vi "Enum To String Method.vi"() -> ()   [LabVIEW 2020]
uses:
  <userlib>/_NEVSTOP/Communicable State Machine(CSM)/_Support/Typedef/_CSM_GlobalLog_MSG_TYPE.ctl
  <userlib>/_NEVSTOP/Communicable State Machine(CSM)/Communicable State Machine.lvlib
panel:
  out "inside 3":i32=999
  out "inside 2":i32=999
  out "inside":i32=999
  out "outside":i32=199
  out "unit (ms)":dbl[][](graph)=[[0.0, 0.0, 0.0, 0.0, 0.0, 0.0, 0.0, 0.0, 0.0, 0.0, 0.0, 0.0, 0.0, 0.0, 0.0, 0.0, 0.0, 0.0, 0.0, 0.0, 0.0, 0.0, 0.0, 0.0, 0.0, 0.0, 0.0, 0.0, 0.0, 0.0, 0.0, 0.0, 0.0, 0.0, 0.0, 0.0, 0.0, 0.0, 0.0, 0.001, 0.0, 0.001, 0.0, 0.0, 0.0, 0.0, 0.0, 0.001, 0.0, 0.0, 0.0, 0.0, 0.0, 0.0, 0.0, 0.0, 0.0, 0.0, 0.0, 0.0, 0.0, 0.0, 0.0, 0.0, 0.0, 0.0, 0.0, 0.0, 0.0, 0.001, 0.0, 0.0, 0.0, 0.0, 0.0, 0.0, 0.0, 0.0, 0.0, 0.0, 0.0, 0.0, 0.0, 0.0, 0.0, 0.0, 0.0, 0.0, 0.0, 0.0, 0.0, 0.0, 0.0, 0.0, 0.001, 0.0, 0.0, 0.0, 0.0, 0.0, 0.0, 0.0, 0.0, 0.0, 0.0, 0.0, 0.0, 0.0, 0.0, 0.0, 0.0, 0.0, 0.0, 0.0, 0.0, 0.0, 0.0, 0.001, 0.0, 0.0, 0.0, 0.0, 0.0, 0.0, 0.001, 0.0, 0.0, 0.0, 0.0, 0.0, 0.0, 0.0, 0.0, 0.0, 0.0, 0.0, 0.0, 0.0, 0.0, 0.0, 0.0, 0.001, 0.0, 0.0, 0.0, 0.0, 0.0, 0.0, 0.0, 0.0, 0.0, 0.0, 0.0, 0.0, 0.0, 0.0, 0.0, 0.0, 0.0, 0.0, 0.0, 0.0, 0.0, 0.0, 0.0, 0.001, 0.001, 0.001, 0.0, 0.0, 0.0, 0.0, 0.0, 0.0, 0.0, 0.001, 0.0, 0.0, 0.0, 0.0, 0.0, 0.0, 0.0, 0.0, 0.0, 0.0, 0.0, 0.0, 0.0, 0.0, 0.0, 0.0, 0.0, 0.0, 0.0, 0.0, 0.0, 0.0, 0.0, 0.0], [0.024, 0.012, 0.007, 0.009, 0.017, 0.007, 0.007, 0.008, 0.007, 0.017, 0.007, 0.009, 0.007, 0.025, 0.021, 0.021, 0.043, 0.037, 0.019, 0.008, 0.006, 0.007, 0.009, 0.007, 0.009, 0.008, 0.007, 0.008, 0.007, 0.008, 0.007, 0.018, 0.01, 0.008, 0.01, 0.008, 0.008, 0.009, 0.009, 0.007, 0.019, 0.007, 0.011, 0.008, 0.01, 0.009, 0.02, 0.009, 0.008, 0.01, 0.007, 0.013, 0.007, 0.007, 0.007, 0.008, 0.007, 0.02, 0.01, 0.007, 0.008, 0.009, 0.012, 0.007, 0.006, 0.009, 0.01, 0.013, 0.012, 0.013, 0.019, 0.01, 0.017, 0.014, 0.016, 0.039, 0.017, 0.018, 0.01, 0.017, 0.014, 0.028, 0.024, 0.031, 0.022, 0.018, 0.007, 0.022, 0.015, 0.016, 0.015, 0.014, 0.009, 0.013, 0.007, 0.014, 0.013, 0.007, 0.009, 0.009, 0.018, 0.008, 0.008, 0.008, 0.008, 0.009, 0.007, 0.009, 0.011, 0.021, 0.007, 0.012, 0.007, 0.009, 0.008, 0.009, 0.017, 0.009, 0.007, 0.008, 0.008, 0.008, 0.014, 0.008, 0.007, 0.009, 0.008, 0.021, 0.009, 0.018, 0.009, 0.011, 0.008, 0.009, 0.009, 0.008, 0.006, 0.011, 0.021, 0.015, 0.008, 0.017, 0.009, 0.008, 0.015, 0.009, 0.008, 0.007, 0.013, 0.012, 0.012, 0.011, 0.01, 0.01, 0.011, 0.013, 0.016, 0.007, 0.009, 0.008, 0.01, 0.009, 0.007, 0.011, 0.019, 0.009, 0.008, 0.015, 0.011, 0.012, 0.012, 0.009, 0.017, 0.009, 0.007, 0.008, 0.013, 0.012, 0.008, 0.018, 0.009, 0.019, 0.01, 0.015, 0.015, 0.016, 0.008, 0.007, 0.009, 0.017, 0.01, 0.008, 0.01, 0.007, 0.006, 0.007, 0.007, 0.009, 0.008, 0.017], [0.006, 0.003, 0.002, 0.007, 0.002, 0.001, 0.002, 0.002, 0.005, 0.002, 0.002, 0.002, 0.005, 0.002, 0.003, 0.011, 0.005, 0.008, 0.002, 0.002, 0.004, 0.001, 0.002, 0.002, 0.002, 0.001, 0.002, 0.002, 0.002, 0.001, 0.003, 0.003, 0.002, 0.003, 0.002, 0.002, 0.001, 0.002, 0.002, 0.002, 0.002, 0.003, 0.002, 0.001, 0.003, 0.002, 0.002, 0.002, 0.002, 0.003, 0.001, 0.002, 0.002, 0.002, 0.002, 0.002, 0.002, 0.003, 0.003, 0.002, 0.002, 0.006, 0.002, 0.004, 0.003, 0.002, 0.005, 0.003, 0.007, 0.002, 0.004, 0.001, 0.006, 0.008, 0.008, 0.006, 0.003, 0.003, 0.002, 0.004, 0.003, 0.004, 0.006, 0.004, 0.005, 0.002, 0.002, 0.003, 0.002, 0.005, 0.004, 0.002, 0.006, 0.002, 0.003, 0.004, 0.003, 0.002, 0.002, 0.001, 0.003, 0.002, 0.002, 0.002, 0.001, 0.002, 0.002, 0.002, 0.011, 0.002, 0.002, 0.002, 0.003, 0.002, 0.002, 0.001, 0.003, 0.002, 0.002, 0.002, 0.002, 0.007, 0.002, 0.002, 0.002, 0.002, 0.002, 0.004, 0.005, 0.002, 0.003, 0.003, 0.003, 0.002, 0.002, 0.003, 0.003, 0.002, 0.004, 0.002, 0.002, 0.004, 0.002, 0.005, 0.002, 0.002, 0.002, 0.002, 0.005, 0.003, 0.007, 0.002, 0.002, 0.004, 0.002, 0.006, 0.003, 0.002, 0.002, 0.002, 0.002, 0.003, 0.002, 0.002, 0.005, 0.001, 0.005, 0.003, 0.001, 0.008, 0.002, 0.001, 0.004, 0.001, 0.002, 0.002, 0.005, 0.003, 0.002, 0.004, 0.002, 0.004, 0.002, 0.004, 0.007, 0.002, 0.005, 0.002, 0.003, 0.004, 0.002, 0.001, 0.002, 0.003, 0.003, 0.002, 0.001, 0.002, 0.003, 0.003]]
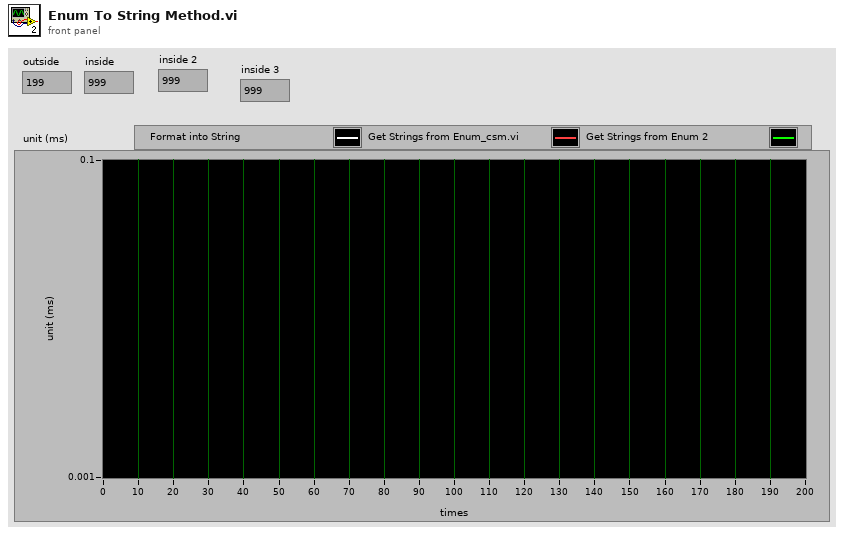
[diagram p1: front panel]
types:
  T1 = typedef "Communicable State Machine.lvlib/_CSM_GlobalLog_MSG_TYPE.ctl" = enum16{"User Log", "State Change", "Status", "Interrupt", "Register", "Unregister", "Error Log", "Module Created", "Module Destroyed"}
  T2 = cluster{"length":u16, "private":u8, "type":enum8{"<Null>", "I8", "I16", "I32", "I64", "U8", "U16", "U32", "U64", "SGL", "DBL", "EXT", "CSG", "CDB", "CXT", "0x0F", "0x10", "0x11", "0x12", "0x13", "0x14", "Enum U8", "Enum U16", "Enum U32", "Enum U64", "SGL PQ", "DBL PQ", "EXT PQ", "CSG PQ", "CDB PQ", "CXT PQ", "0x1F", "0x20", "Boolean", "0x22", "0x23", "0x24", "0x25", "0x26", "0x27", "0x28", "0x29", "0x2A", "0x2B", "0x2C", "0x2D", "0x2E", "0x2F", "String", "0x31", "Path", "Pict", "0x34", "0x35", "0x36", "DAQ", "0x38", "0x39", "0x3A", "0x3B", "0x3C", "0x3D", "0x3E", "0x3F", "Array", "0x41", "0x42", "0x43", "0x44", "0x45", "0x46", "0x47", "0x48", "0x49", "0x4A", "0x4B", "0x4C", "0x4D", "0x4E", "0x4F", "Cluster", "0x51", "0x52", "Variant", "Waveform", "0x55", "0x56", "0x57", "0x58", "0x59", "0x5A", "0x5B", "0x5C", "0x5D", "0x5E", "Fixed Point", "0x60", "0x61", "0x62", "0x63", "0x64", "0x65", "0x66", "0x67", "0x68", "0x69", "0x6A", "0x6B", "0x6C", "0x6D", "0x6E", "0x6F", "Refnum", "0x71", "0x72", "Set Collection", "Map Collection"}, "# elements":u16}
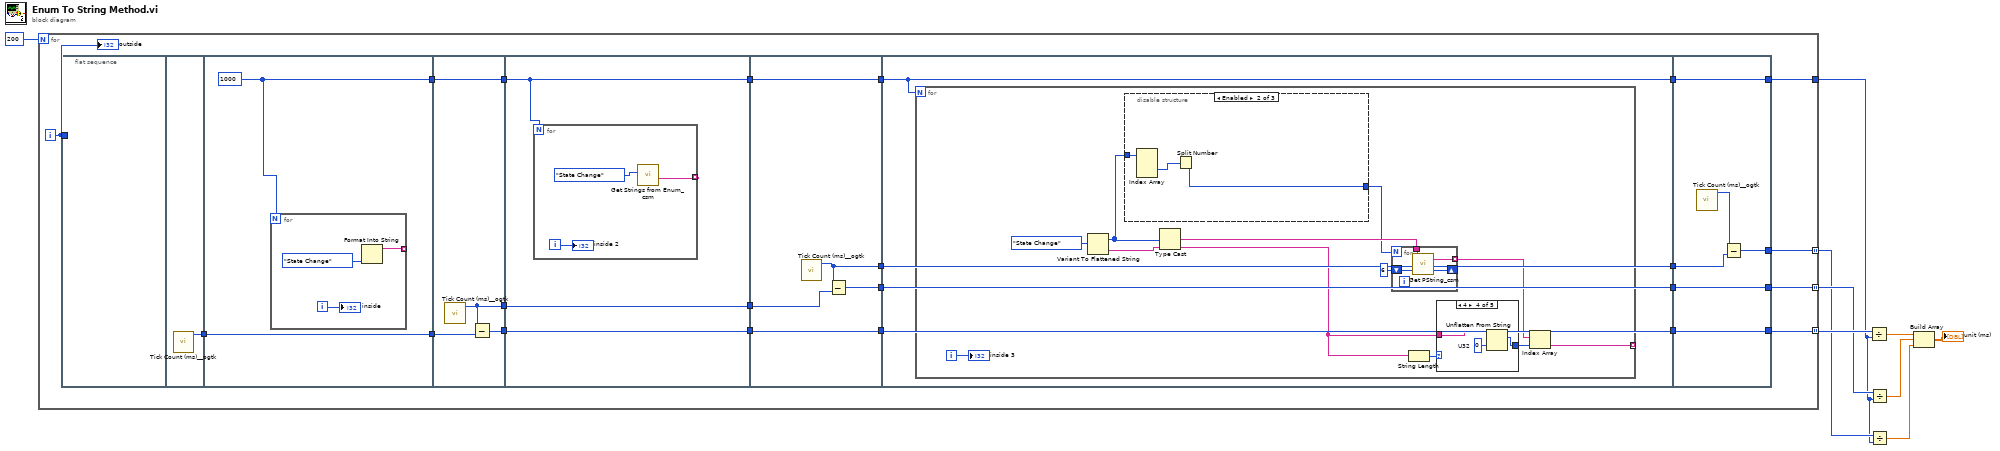
[diagram p0: block diagram]
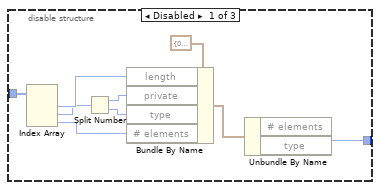
[diagram p2: hidden frame]
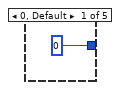
[diagram p4: hidden frame]
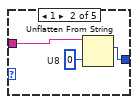
[diagram p5: hidden frame]
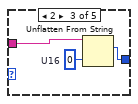
[diagram p6: hidden frame]
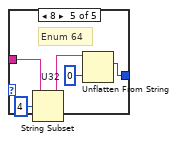
[diagram p7: hidden frame]
diagram:
  n1 = for {
    N: 200 -> [_]
    tunnel: [w29] -> w9 mode=indexing
    tunnel: [w28] -> w2
    tunnel: [w19] -> w5 mode=indexing
    tunnel: [w10] -> w3 mode=indexing
    i -> [w26]
    n2 = flat-sequence {
      tunnel: w26 -> [_]
      tunnel: [w32] -> w31
      tunnel: w31 -> [w34]
      tunnel: [w34] -> w30
      tunnel: [w33] -> w27
      tunnel: w30 -> [w41]
      tunnel: w27 -> [w39]
      tunnel: [w40] -> w25
      tunnel: [w39] -> w24
      tunnel: [w38] -> w20
      tunnel: w25 -> [w44]
      tunnel: w24 -> [w42]
      tunnel: [w44] -> w23
      tunnel: [w42] -> w22
      tunnel: [w43] -> w21
      tunnel: w20 -> [w43]
      tunnel: w23 -> [w52]
      tunnel: w22 -> [w51]
      tunnel: w21 -> [w50]
      tunnel: [w52] -> w18
      tunnel: [w51] -> w17
      tunnel: [w49] -> w16
      tunnel: [w48] -> w12
      tunnel: w18 -> [w56]
      tunnel: w17 -> [w53]
      tunnel: w16 -> [w55]
      tunnel: [w56] -> w15
      tunnel: [w53] -> w14
      tunnel: [w55] -> w13
      tunnel: w12 -> [w54]
      tunnel: [w54] -> w11
      tunnel: [w102] -> w19
      tunnel: [w103] -> w28
      tunnel: [w104] -> w29
      tunnel: w15 -> [w104]
      tunnel: w14 -> [w103]
      tunnel: w13 -> [w102]
      tunnel: w11 -> [w100]
      tunnel: [w99] -> w10
      frame #0 {
      }
      frame #1 {
        n3 = call <userlib>:"Tick Count (ms)__ogtk.vi"() -> ("millisecond timer value"=w32:u32)  [unwired: 10 in, 1 out]
      }
      frame #2 {
        w33 = 1000
        n4 = for {
          N: w33 -> [_]
          tunnel: [w35] -> _ mode=indexing
          i -> [w37]
          n5 = Format Into String(_CSM_GlobalLog_MSG_TYPE."State Change" ("LogType")) -> (resulting string=w35:string)  [unwired: 3 in, 1 out]
          "inside" <- w37
        }
      }
      frame #3 {
        n6 = call <userlib>:"Tick Count (ms)__ogtk.vi"() -> ("millisecond timer value"=w38:u32)  [unwired: 10 in, 1 out]
        n7 = Subtract(x=w38, y=w41) -> (x-y=w40:u32)
      }
      frame #4 {
        n8 = for {
          N: w42 -> [_]
          tunnel: [w45] -> _ mode=indexing
          i -> [w47]
          n9 = call <userlib>:"Get Strings from Enum_csm.vi"("Enum"=_CSM_GlobalLog_MSG_TYPE."State Change" ("LogType")) -> ("String Value"=w45:string)  [unwired: 7 in, 3 out]
          "inside 2" <- w47
        }
      }
      frame #5 {
        n10 = call <userlib>:"Tick Count (ms)__ogtk.vi"() -> ("millisecond timer value"=w48:u32)  [unwired: 10 in, 1 out]
        n11 = Subtract(x=w48, y=w50) -> (x-y=w49:u32)
      }
      frame #6 {
        n12 = for {
          N: w53 -> [_]
          tunnel: [w57] -> _ mode=indexing
          i -> [w67]
          n13 = Variant To Flattened String(Variant=_CSM_GlobalLog_MSG_TYPE."State Change" ("LogType")) -> (data string=w61:string, 1:w60:i16[])
          n14 = disable-structure shown="Enabled" {
            disable-tunnel: [w76 w77 _] -> w63
            disable-tunnel: w60 -> [w70 w78 _]
            frame Disabled {
              n15 = Index Array(array=w70) -> (element #1=w75:i16, element #2=w72:i16, element #3=w71:i16)  [unwired: 3 in]
              n16 = Split Number(x=w72) -> (hi(x)=w74:u8, lo(x)=w73:u8)
              n17 = Bundle By Name(cluster=T2 {"length"=0, "private"=0, "type"=enum."<Null>", "# elements"=0} ("Type Descriptor Header"), "length"=w75, "private"=w74, "type"=w73, "# elements"=w71) -> (w69:T2)
              n18 = Unbundle By Name(w69) -> ("# elements"=w76:u16)  [unwired: 1 out]
            }
            frame Enabled {
              n19 = Index Array(array=w78) -> (element #2=w79:i16)  [unwired: 3 in, 2 out]
              n20 = Split Number(x=w79) -> (lo(x)=w77:u8)  [unwired: 1 out]
            }
            frame Disabled {
            }
          }
          n21 = Type Cast(x=w60) -> (*(type *) &x=w66:string)  [unwired: 1 in]
          n22 = for {
            N: w63 -> [_]
            tunnel: w66 -> [w80]
            shift-right: [w81] -> _
            shift-left: 6 -> [w82]
            tunnel: [w83] -> w62 mode=indexing
            n23 = call <userlib>:"Get PString_csm.vi"("offset (0)"=w82, "String"=w80) -> ("offset past PString"=w81:i32, "PString"=w83:string)
          }
          n24 = String Length(string=w61) -> (length=w64:i32)
          n25 = case shown="4" w64 {
            tunnel: w61 -> [_ w87 w90 w93 w94]
            tunnel: [u32 0 ("U32") w85 w88 w91 w97] -> w65
            frame 0, Default {
            }
            frame 1 {
              w86 = u8 0  # U8
              n26 = Unflatten From String(type=w86, binary string=w87) -> (value=w85:u8)  [unwired: 3 in, 2 out]
            }
            frame 2 {
              w89 = u16 0  # U16
              n27 = Unflatten From String(type=w89, binary string=w90) -> (value=w88:u16)  [unwired: 3 in, 2 out]
            }
            frame 4 {
              w92 = u32 0  # U32
              n28 = Unflatten From String(type=w92, binary string=w93) -> (value=w91:u32)  [unwired: 3 in, 2 out]
            }
            frame 8 {
              w98 = u32 0  # U32
              # "Coerce Data to U32"
              # "Enum 64"
              n29 = String Subset(string=w94, offset (0)=4) -> (substring=w95:string)  [unwired: 1 in]
              n30 = Unflatten From String(type=w98, binary string=w95) -> (value=w97:u32)  [unwired: 3 in, 2 out]
            }
          }
          n31 = Index Array(array=w62, index=w65) -> (element=w57:string)
          "inside 3" <- w67
        }
      }
      frame #7 {
        n32 = call <userlib>:"Tick Count (ms)__ogtk.vi"() -> ("millisecond timer value"=w101:u32)  [unwired: 10 in, 1 out]
        n33 = Subtract(x=w101, y=w100) -> (x-y=w99:u32)
      }
    }
    "outside" <- w26
  }
  n34 = Divide(x=w9, y=w2) -> (x/y=w6:dbl[])
  n35 = Divide(x=w5, y=w2) -> (x/y=w4:dbl[])
  n36 = Divide(x=w3, y=w2) -> (x/y=w1:dbl[])
  n37 = Build Array(w6, w4, w1) -> (→"unit (ms)":dbl[][])
